vi "MakePacket.vi"(8 "error in (no error)":errorcluster, 10 "Data":string, 11 "STATE":string) -> (0 "error out":errorcluster, 3 "<JSON>":string)   [LabVIEW 2020]
uses:
  981bfa90-5ea9-4df4-96dc-1f9857a92501.vi
  <vilib>/JDP Science/JSONtext/Variant to JSON Text.vi
  <vilib>/JDP Science/JSONtext/JSONtext.lvlib
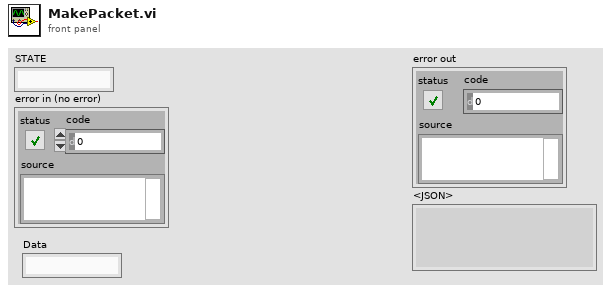
[diagram p1: front panel]
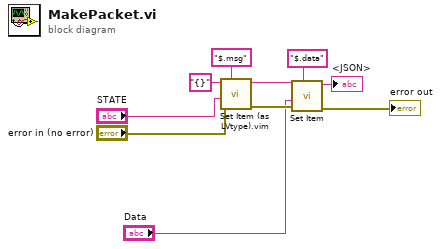
[diagram p0: block diagram]
diagram:
  n1 = call "Set Item (as LVtype).vim"("Object (or Item) Path"="$.msg" ("$Path or Item Name"), "error in (no error)"="error in (no error)", "Anything"="STATE", "JSON"="{}") -> ("error out"=w4:errorcluster, "<JSON>"=w7:string)  [unwired: 4 in, 1 out]
  n2 = call <vilib>:"Set Item.vi"("$Path or Item Name"="$.data", "error in (no error)"=w4, "JSON to Insert"="Data", "JSON"=w7) -> ("error out"=→"error out":errorcluster, "<JSON>"=→"<JSON>":string)  [unwired: 4 in, 1 out]
